vi "bin to string.vi"(10 "Data in":u8[](array[numeric]) format="%.0x") -> (2 "string":string)   [LabVIEW 2018, in "EF20.lvlib" / "EF20.lvclass"]
uses:
  EF20.lvclass
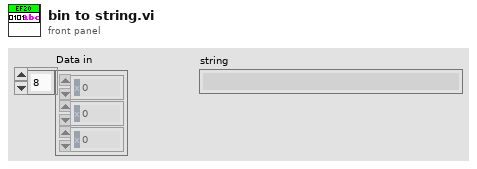
[diagram p1: front panel]
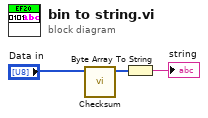
[diagram p0: block diagram]
diagram:
  n1 = call "Checksum.vi"("Data In"="Data in") -> ("Data with Cksum"=w1:u8[])  [unwired: 9 in, 1 out]
  n2 = Byte Array To String(unsigned byte array=w1) -> (string=→"string":string)
